vi "Write Listener Settings.vi"(8 "error in (no error)":errorcluster, 10 "Listener Settings":T1={"resolve remote address (T)"=TRUE, "timeout ms (-1)"=0, "net address"=0, "port"=0}, 11 "WebSocket Server in":refnum<class "WebSocket Server.lvclass">) -> (0 "error out":errorcluster, 3 "WebSocket Server out":refnum<class "WebSocket Server.lvclass">)   [LabVIEW 2016, in "WebSocket Actor.lvlib" / "WebSocket Server.lvclass"]
uses:
  WebSocket Server.lvclass
  typedefs/Listener Settings.ctl
  WebSocket Server.lvclass/WebSocket Server.ctl
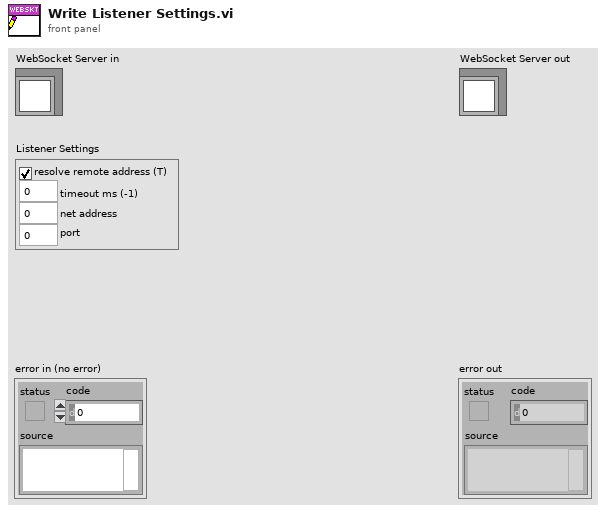
[diagram p1: front panel]
types:
  T1 = typedef "WebSocket Actor.lvlib/WebSocket Server.lvclass/Listener Settings.ctl" = cluster{"resolve remote address (T)":bool, "timeout ms (-1)":i32, "net address":u32, "port":u16}
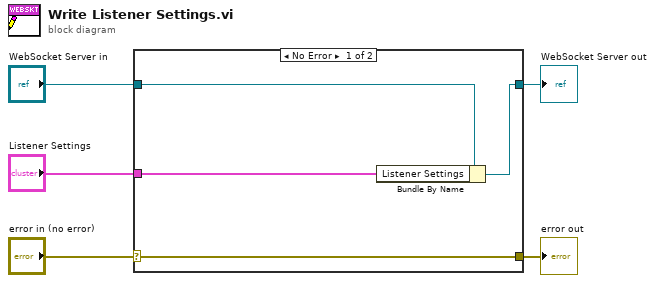
[diagram p0: block diagram]
diagram:
  n1 = case shown="No Error" "error in (no error)" {
    selector: "error in (no error)" -> [w9 w10]
    tunnel: [w9 w10] -> w4
    tunnel: [w7 w11] -> w2
    tunnel: "WebSocket Server in" -> [w8 w11]
    tunnel: "Listener Settings" -> [w6 _]
    frame No Error {
      n2 = Bundle By Name(cluster=w8, "Listener Settings"=w6) -> (w7:refnum<class "WebSocket Server.lvclass">)
    }
    frame Error {
    }
  }
  "error out" <- w4
  "WebSocket Server out" <- w2
